vi "subscribe.vi"(8 "error in (no error)":errorcluster, 10 "source":string, 11 "ActiveMQBroker in":refnum<class "ActiveMQBroker.lvclass">) -> (0 "error out":errorcluster, 3 "ActiveMQBroker out":refnum<class "ActiveMQBroker.lvclass">)   [LabVIEW 2024, in "ActiveMQBroker.lvclass"]
uses:
  ActiveMQBroker.lvclass
  ActiveMQBroker.lvclass/ActiveMQBroker.ctl
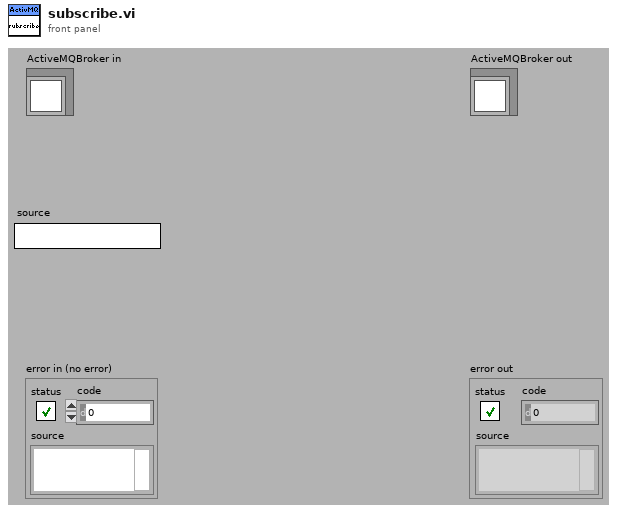
[diagram p1: front panel]
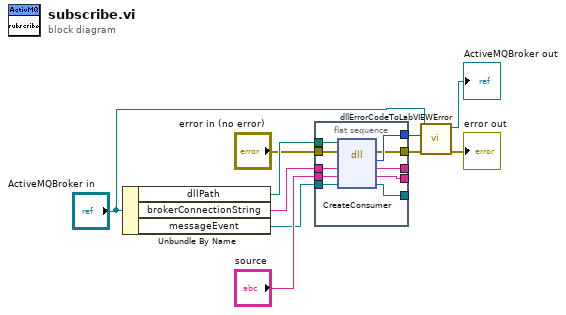
[diagram p0: block diagram]
diagram:
  n1 = Unbundle By Name("ActiveMQBroker in") -> ("dllPath"=w10:path, "brokerConnectionString"=w8:string, "messageEvent"=w6:refnum<user-event>)
  n2 = flat-sequence {
    tunnel: w10 -> [w20]
    tunnel: "error in (no error)" -> [w19]
    tunnel: w8 -> [w18]
    tunnel: "source" -> [w17]
    tunnel: w6 -> [w16]
    tunnel: [w15] -> w5
    tunnel: [w14] -> w4
    tunnel: [w13] -> _
    tunnel: [w12] -> _
    tunnel: [w11] -> _
    frame #0 {
      n3 = dll-call lib="?" fn="CreateConsumer"(path in=w20, error in=w19, "brokerURI"=w18, "topicName"=w17, "event"=w16) -> (error out=w14:errorcluster, "consumerID"=w15:u32, "brokerURI"=w13:string, "topicName"=w12:string, "event"=w11:refnum<user-event>)  [unwired: 1 in, 1 out]
    }
  }
  n4 = call "dllErrorCodeToLabVIEWError.vi"("error in (no error)"=w4, "error code in"=w5, "ActiveMQBroker in"="ActiveMQBroker in") -> ("error out"=→"error out":errorcluster, "ActiveMQBroker out"=→"ActiveMQBroker out":refnum<class "ActiveMQBroker.lvclass">)  [unwired: 7 in]
